vi "Pack to Any.vi"(8 "error in":errorcluster, 9 "data to pack":T1, 10 "message type":string, 11 "gRPC ID in":T2) -> (0 "error out":errorcluster, 2 "any":T3, 3 "gRPC ID out":T2)   [LabVIEW 2020, in "Client.lvlib"]
uses:
  Client/Client.lvlib
  <vilib>/gRPC/LabVIEW gRPC Library/Shared/grpcId.ctl
  <vilib>/gRPC/LabVIEW gRPC Library/Shared/Any.ctl
  <vilib>/AdvancedString/1D String Array to Delimited String.vi
  <vilib>/gRPC/LabVIEW gRPC Library/grpc-lvsupport-release.lvlib
  Service/Service/Measurement Configuration.ctl
  Service/Service/Service.lvlib
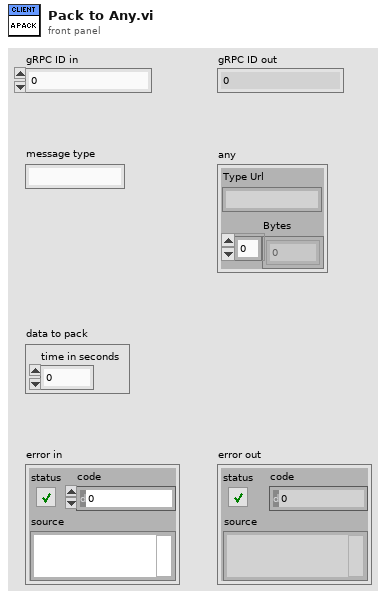
[diagram p1: front panel]
types:
  T1 = typedef "Service.lvlib/Measurement Configuration.ctl" = cluster{"time in seconds":dbl}
  T2 = typedef "grpc-lvsupport-release.lvlib/grpcId.ctl" = u64
  T3 = typedef "grpc-lvsupport-release.lvlib/Any.ctl" = cluster{"Type Url":string, "Bytes":u8[]}
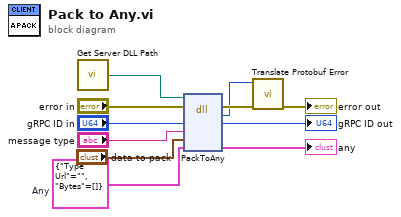
[diagram p0: block diagram]
diagram:
  w6 = T3 {"Type Url"="", "Bytes"=[]}  # Any
  n1 = call <vilib>:"Get Server DLL Path.vi"() -> ("Server dll path"=w9:path)
  n2 = dll-call lib="?" fn="PackToAny"(path in=w9, error in="error in", "gRPCId"="gRPC ID in", "messageType"="message type", "value"="data to pack", "any"=w6) -> (error out=w10:errorcluster, "return type"=w3:i32, "gRPCId"=→"gRPC ID out":u64, "any"=→"any":T3)  [unwired: 3 in, 1 out]
  n3 = call <vilib>:"Translate Protobuf Error.vi"("error in"=w10, "Error Code"=w3) -> ("error out"=→"error out":errorcluster)  [unwired: 9 in]
